vi "Result_Test.vi"(8 "error in (no error)":errorcluster caption="entrée d'erreur (pas d'erreur)", 11 "Delay en entrée":refnum<class "Wait_Voltage.lvclass">) -> (0 "error out":errorcluster caption="sortie d'erreur", 3 "Delay en sortie":refnum<class "Wait_Voltage.lvclass">)   [LabVIEW 2020, in "Library Test.lvlib" / "Wait_Voltage.lvclass"]
uses:
  Wait_Voltage.lvclass
  C:/Users/ngarcin/OneDrive - Altyor/Standard TB/Class/Test/Test (Default)/Test (Default).lvclass
  Test_Without_Instr/Test_Without_Inst.lvclass
  Wait_Voltage.lvclass/Wait_Voltage.ctl
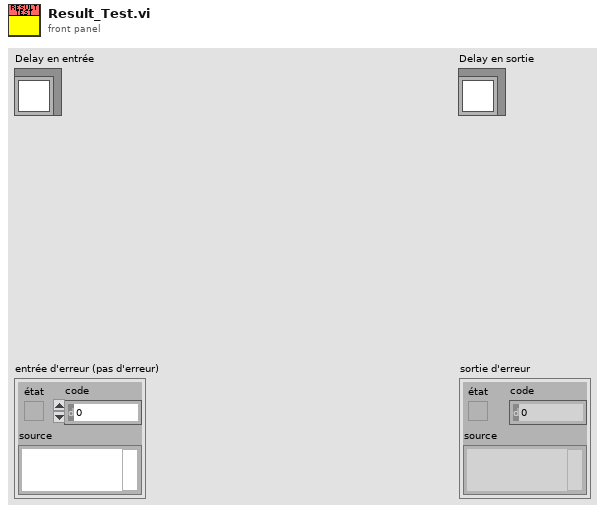
[diagram p1: front panel]
types:
  T1 = enum16{"Get Variable", "Get All Variables", "Set Variable", "Delete Variable", "Delete All Variable"}
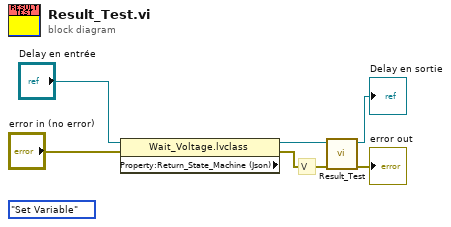
[diagram p0: block diagram]
diagram:
  (unwired) T1."Set Variable" ("Function")
  # "V"
  n1 = property class="Wait_Voltage.lvclass" props=["Property:Return_State_Machine (Json)"](reference="Delay en entrée", error in="error in (no error)") -> (reference out=w3:refnum<class "Wait_Voltage.lvclass">, error out=w1:errorcluster)  [unwired: 1 out]
  n2 = call-parent "Result_Test.vi"("error in (no error)"=w1, "Test_Without_Inst en entrée"=w3) -> ("error out"=→"error out":errorcluster, "Test_Without_Inst en sortie"=→"Delay en sortie":refnum<class "Wait_Voltage.lvclass">)  [unwired: 8 in]
